vi "Property_Always Refresh.vi"(8 "error in (no error)":errorcluster, 11 "Dependency Source in":refnum<class "Dependency Source.lvclass">) -> (0 "error out":errorcluster, 2 "Always Refresh Targets?":bool, 3 "Dependency Source out":refnum<class "Dependency Source.lvclass">)   [LabVIEW 2019, in "Project.Dependencies Finder.lvlib" / "Dependency Source.lvclass"]
doc: "Set this property to override the refresh behaviour. If True the Dependency Source will be skipped on 'Refresh Target' but always refreshed when finding dependencies.\n\nThe default implementation returns False."
uses:
  Dependency Source.lvclass
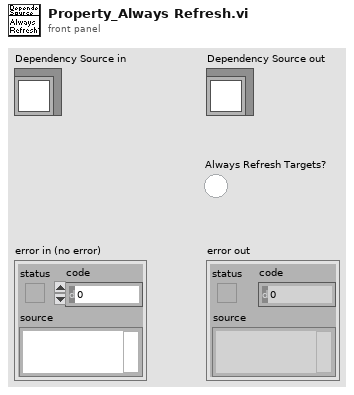
[diagram p1: front panel]
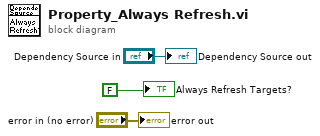
[diagram p0: block diagram]
diagram:
  "error out" <- "error in (no error)"
  "Dependency Source out" <- "Dependency Source in"
  "Always Refresh Targets?" <- FALSE
